vi "Dashboard Main.vi"() -> ()   [LabVIEW 2015]
uses:
  <vilib>/Utility/miscctls.llb/LVRowAndColumnTypeDef.ctl
  <vilib>/event_ctls.llb/eventvkey.ctl
  <vilib>/Rock Robotics/WPI/Dashboard/WPI_DashboardLogging Global.vi
  <vilib>/Utility/config.llb/Write Key (String).vi
  <vilib>/Utility/config.llb/Write Key (I32).vi
  <vilib>/Utility/config.llb/NI_LVConfig.lvlib
panel:
  in  "TCP":refnum<k5>
  in  "Rec Mode":enum32{"Stop", "Record", "Playback"}(radio)
  in  "Vision":u16(ring) items=["Camera Off", "USB Camera SW", "USB Camera HW", "IP Camera"]
  out "Camera IP":string
  out "Image Message":string="Timeout in Camera Communications"
  in  "Dashboard Tab":T1(tab)
  out "Velocity":dbl
  out "Centered":bool
  out "Can Hit":bool
  out "Visable Image":bool
  out "Can Fit":bool
  out "Posible Velocity":bool
  out "MotorSlide4 2":dbl(slide) scale=0.0..14.0 scale format="%#_2e"
  in  "Select Auto":string(combo)
  out "NT Connection":bool
  in  "Camera Settings":T2={"Frame Rate"=30, "Compression"=30, "Size"=1} {"Frame Rate" scale=1.0..30.0; "Size" items=["640x480", "320x240", "160x120"]}
  out "Battery":cluster{"Battery V":dbl}(graph)
  out "Mode":T3(ring)=enum."Auto Disabled"
  in  "DB Camera Config":bool
  out "fps":dbl format="%#.1g"
  out "Mbps":dbl format="%#.1g"
  out "Mbps LED":bool
  in  "Test Slider":dbl(slide) scale=0.0..100.0 scale format="%#_3g"
  in  "On/Off":bool caption="Solenoid"
  in  "Test Name":u16(ring) items=["Select the test to run..."]
  in  "Test Tree":string(tree)
  in  "Motor":cluster{"Value":dbl, "Enable":bool} {"Value" scale=-1.0..1.0 scale format="%#_3g"}
  out "Progress":T4 {"Test Progress" scale=0.0..100.0}
  in  "Rev/Fwd":cluster{"Forward":bool, "Reverse":bool}
  in  "Test Ring":u16(ring) items=["Monochrome", "Color"]
  out "Cmd Status":string
  in  "Execute Command":bool
  in  "Command Params":string[][](table)
  in  "Command Selection":i32(listbox)
  in  "CheckList":i32(listbox)=11
  out "Tree":string(tree)
  out "Camera Image":T5(plugin-control)
  out "Background":bool
  # "Battery"
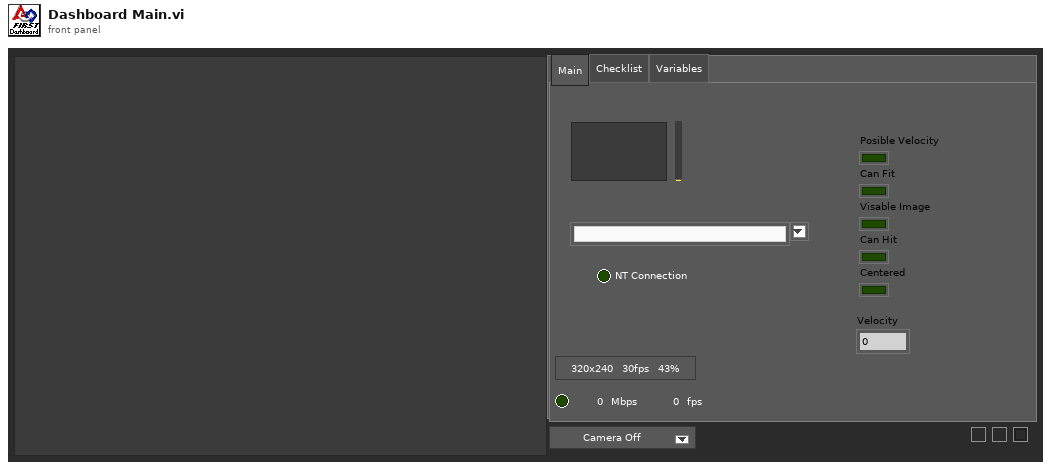
[diagram p1: front panel]
types:
  T1 = enum32{"Main", "Test", "Commands", "Checklist", "Variables"}
  T2 = cluster{"Frame Rate":i32, "Compression":i32, "Size":u16}
  T3 = enum8{"Tele-Op Disabled", "Tele-Op Enabled", "Auto Disabled", "Auto Enabled", "Test Disabled", "Test Enabled", "Disconnected", "No Code", "E-Stop"}
  T4 = cluster{"Test Progress":u8, "Test Progress Text":string}
  T5 = typedef "IMAQ Image.ctl" = refnum<image>
  T6 = cluster{"IDs":cluster{"RPC field ID":u16, "Unique ID":u16}, "String":string}
  T7 = enum32{"Drive", "Basic", "Custom", "Test", "Checklist", "Variables"}
  T8 = typedef "Image Type" = u32
  T9 = cluster{"Camera Image":refnum<vi>, "Dashboard Tab":refnum<vi>, "Background":refnum<vi>, "Vision":refnum<vi>, "Rec Mode":refnum<vi>, "Test Slider":refnum<vi>, "On/Off ":refnum<vi>, "Test Ring":refnum<vi>, "Rev/Fwd":refnum<vi>, "Test Name":refnum<vi>, "Motor":refnum<vi>, "Progress":refnum<vi>, "CheckList":refnum<vi>, "Tree":refnum<vi>, "Test Tree":refnum<vi>, "Command Params":refnum<vi>, "Command Selection":refnum<vi>, "Execute Command":refnum<vi>, "Cmd Status":refnum<vi>}
  T10 = cluster{"Error Strings":string, "Disable Counts":cluster{u16, u16}, "Rail Faults":cluster{u16, u16, u16}, "Robot IP":string, "DB Mode":u8, "Event Info":cluster{"Name":string, "Type":u8, "Number":u16, "Replay":u8}, "Camera Addr":string}
  T11 = cluster{"Status bits":cluster{"Test Mode":bool, "Autonomous":bool, "Enabled":bool, "Code Start":bool, "Brownout":bool, "Reserved 2":bool, "Reserved 3":bool, "E-Stop":bool}, "Code Trace":cluster{"Disabled":bool, "TeleOp":bool, "Auto":bool, "Test":bool}, "Controller Type":enum16{"unknown", "cRIO", "roboRio"}, "Code?":enum16{"unknown", "noCode", "code"}, "Battery V":dbl}
  T12 = cluster{"Control Bits":cluster{"TestMode":bool, "Autonomous":bool, "Enabled":bool, "FMS Present":bool, bool, bool, bool, "E-Stop":bool}, "Team Station ":u8, "Countdown":sgl, "Joystick Values":cluster{"Axes":dbl[], "Buttons":bool[], "POVs":i16[]}[]}
  T13 = typedef "NI_LVConfig.lvlib/Config Data RefNum.ctl" = refnum<k1>
  T14 = cluster{"Operation":enum16{"Update", "Clear"}, "Color Box":u32}[]
  T15 = typedef "eventvkey.ctl" = enum16{"ASCII", "Enter", "Return", "Shift", "Ctrl", "Alt", "Cmd", "Opt", "Caps", "NumLock", "Clear", "Break", "Up", "Down", "Left", "Right", "Insert", "Delete", "Home", "End", "PageUp", "PageDown", "Escape", "Help", "Pause", "ScrollLock", "F1", "F2", "F3", "F4", "F5", "F6", "F7", "F8", "F9", "F10", "F11", "F12", "F13", "F14", "F15", "F16", "F17", "F18", "F19", "F20", "F21", "F22", "F23", "F24", "Play", "VolumeUp", "VolumeDown", "Mute", "Two Byte Char"}
  T16 = cluster{"Image Size":bool, "Image Type":bool, "Pixel Value":bool, "ROI Information":bool, "Zoom Factor":bool}
  T17 = enum8{"Enabled", "Disabled", "Disabled and Grayed Out"}
  T18 = cluster{"Operation":enum16{"Update", "Clear"}, "Color Box":u32}
  T19 = typedef "LVRowAndColumnTypeDef.ctl" = cluster{"Row":i32, "Column":i32}
  T20 = cluster{"Shift":bool, "Ctrl":bool, "Alt":bool, "Cmd":bool, "Opt":bool}
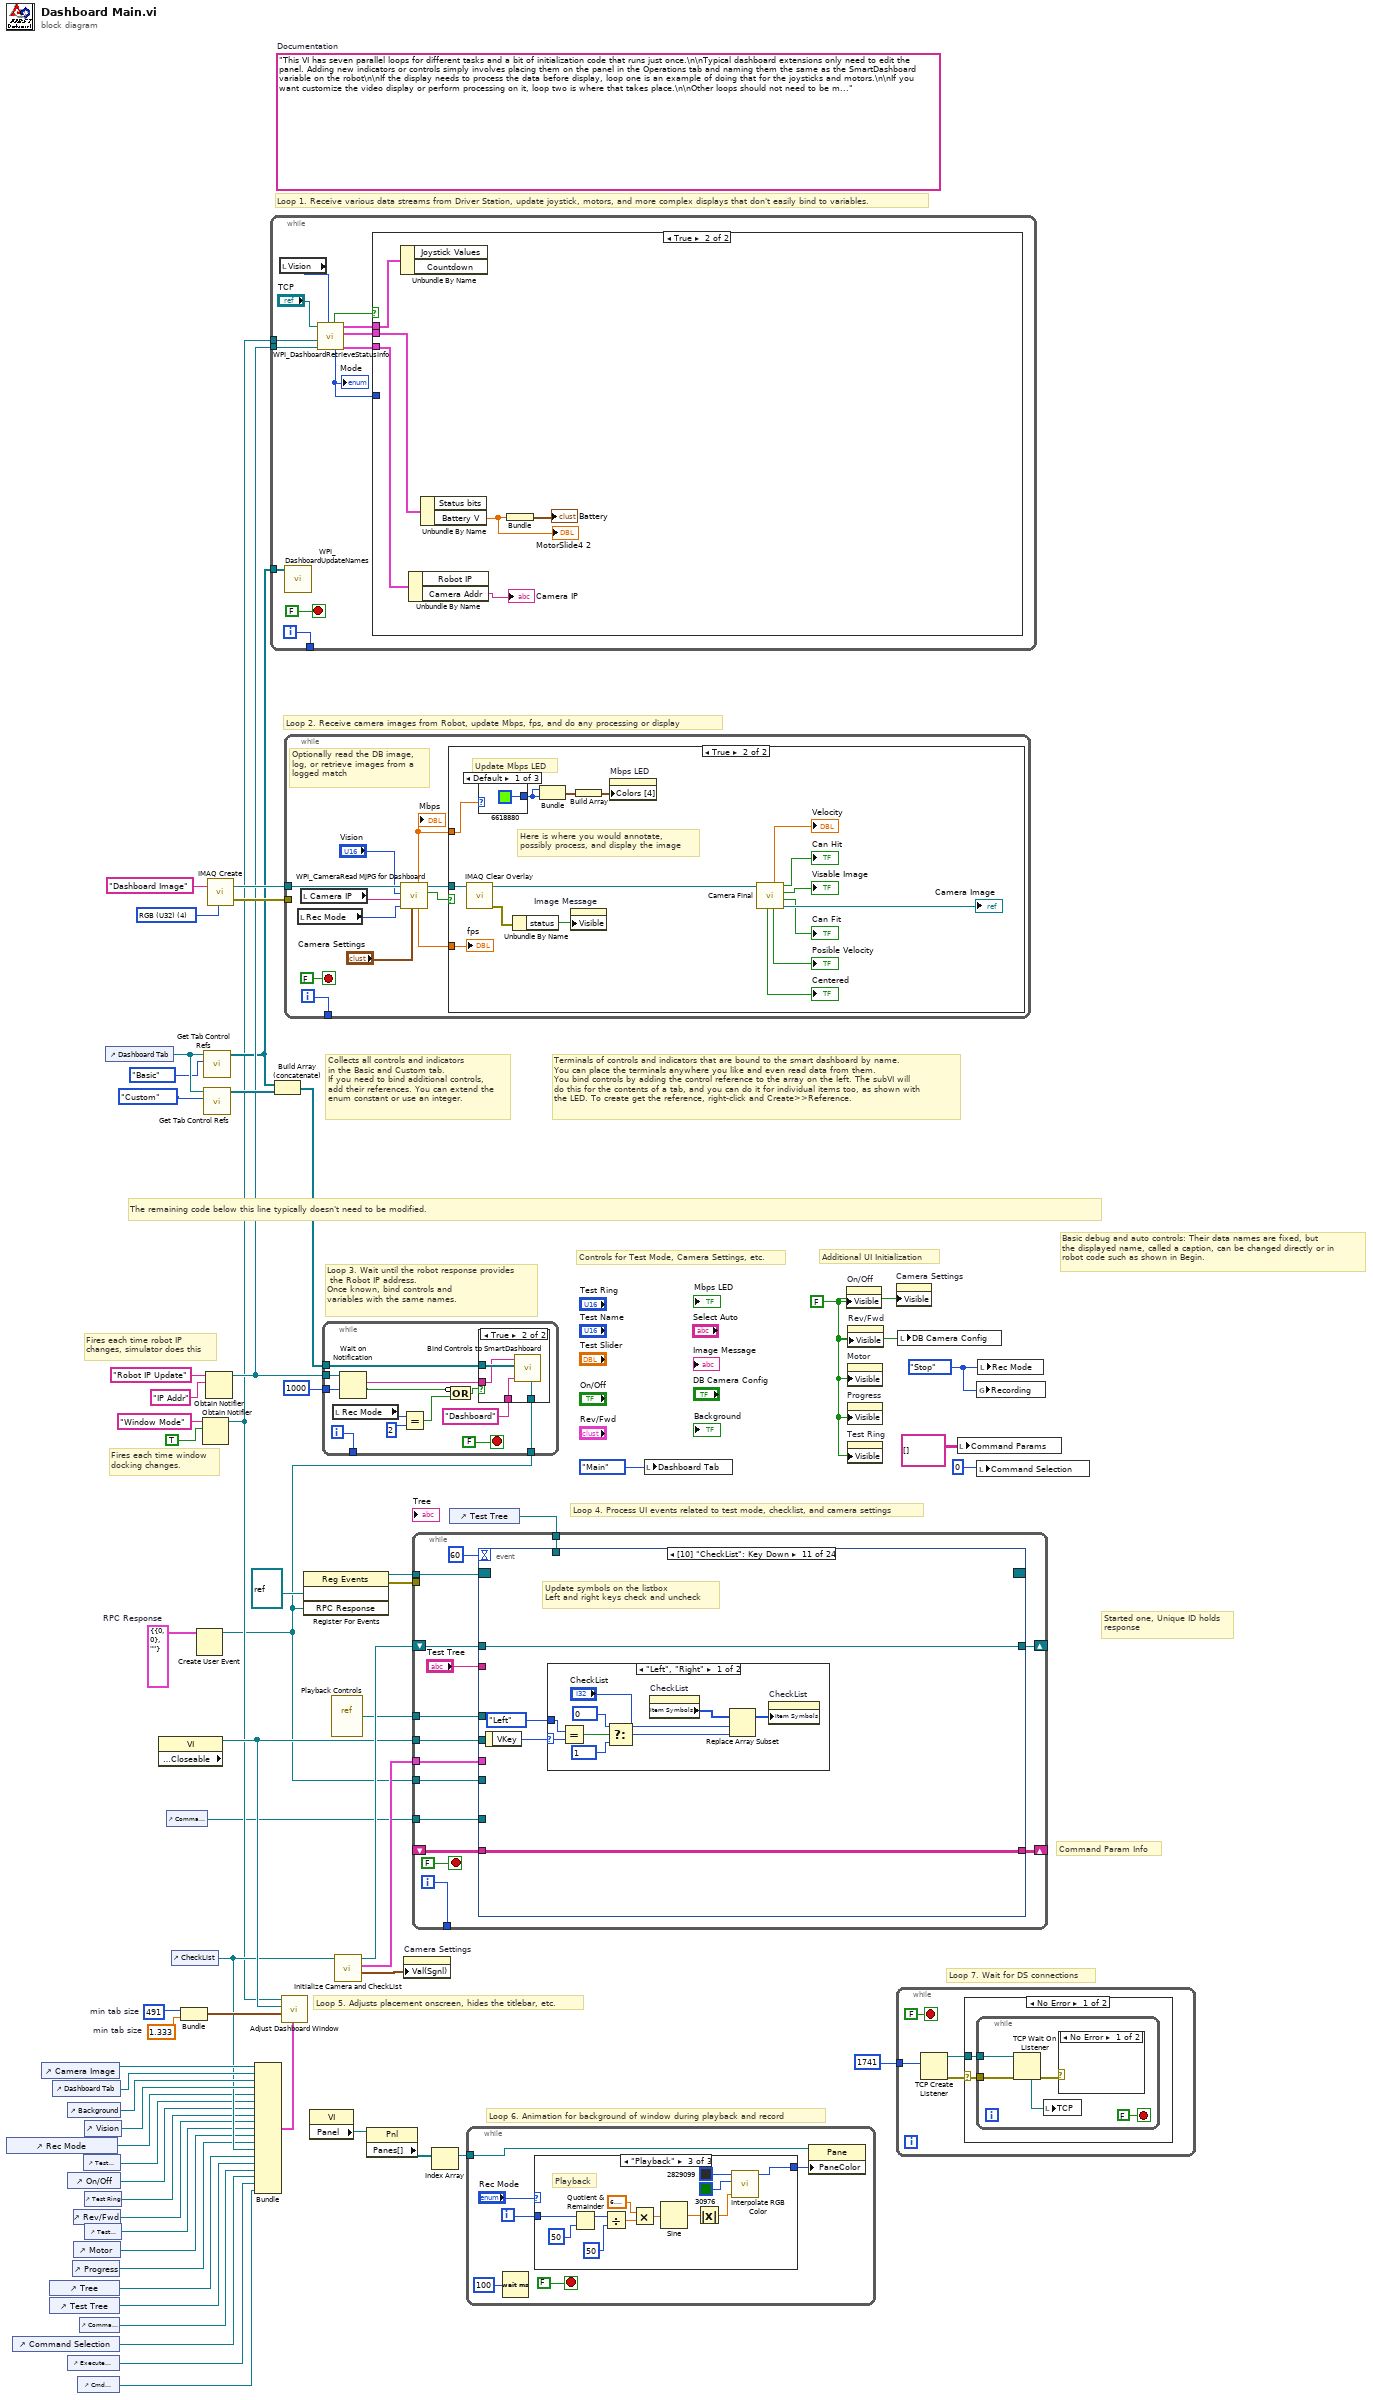
[diagram p0: block diagram]
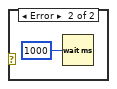
[diagram p2: hidden frame]
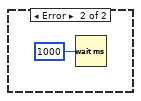
[diagram p3: hidden frame]
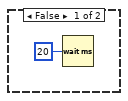
[diagram p4: hidden frame]
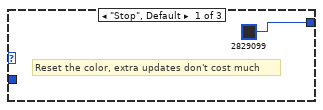
[diagram p5: hidden frame]
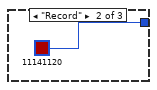
[diagram p6: hidden frame]
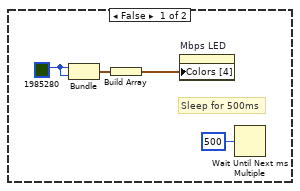
[diagram p8: hidden frame]
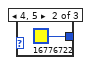
[diagram p9: hidden frame]
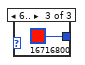
[diagram p10: hidden frame]
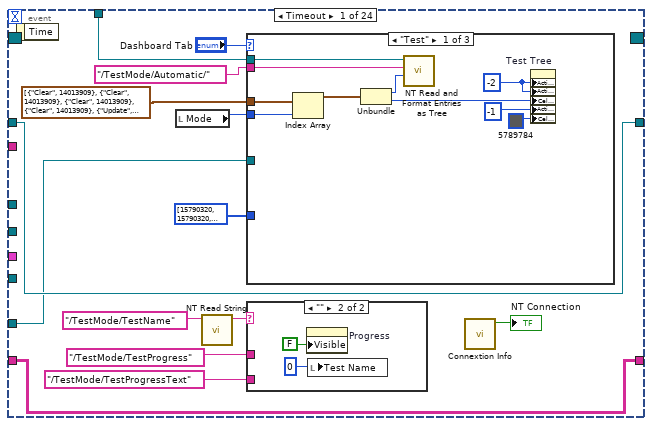
[diagram p11: hidden frame]
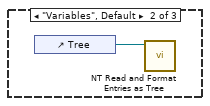
[diagram p12: hidden frame]
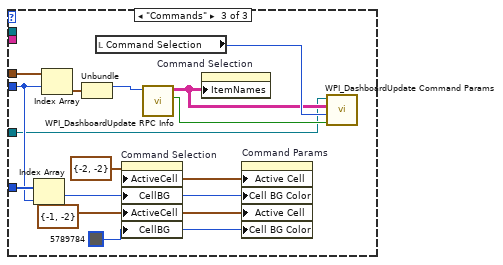
[diagram p13: hidden frame]
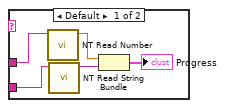
[diagram p14: hidden frame]
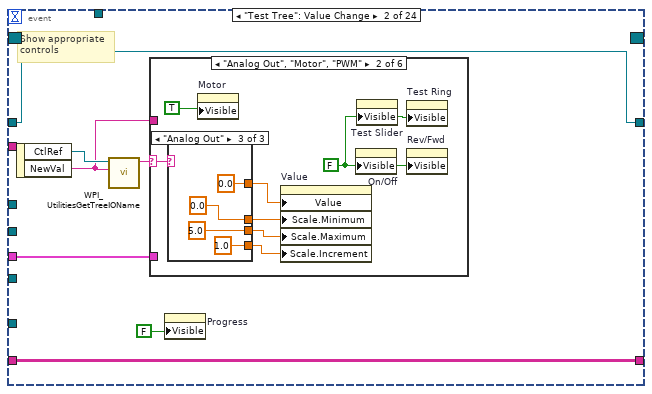
[diagram p15: hidden frame]
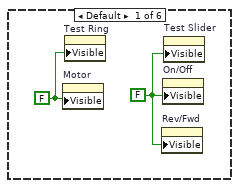
[diagram p16: hidden frame]
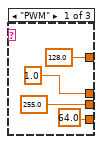
[diagram p17: hidden frame]
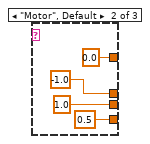
[diagram p18: hidden frame]
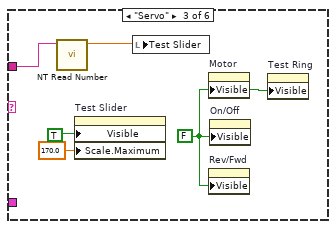
[diagram p19: hidden frame]
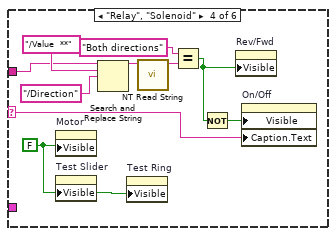
[diagram p20: hidden frame]
diagram:
  w8 = T6 {"IDs"={"RPC field ID"=0, "Unique ID"=0}, "String"=""}  # RPC Response
  w33 = 491  # min tab size
  w32 = 1.333  # min tab size
  w41 = enum32{"Stop", "Record", "Playback"}."Stop" ("Rec Mode")
  w15 = FALSE ("Visible")
  (unwired) "This VI has seven parallel loops for different tasks and a bit of initialization code that runs just once.\n\nTypical dashboard extensions only need to edit the panel. Adding new indicators or controls simply involves placing them on the panel in the Operations tab and naming them the same as the SmartDashboard variable on the robot\n\nIf the display needs to process the data before display, loop one is an example of doing that for the joysticks and motors.\n\nIf you want customize the video display or perform processing on it, loop two is where that takes place.\n\nOther loops should not need to be modified. They are pretty standard, and document the task they perform."  # Documentation
  w61 = T8 4 items=["Grayscale (U8)", "Grayscale (I16)", "Grayscale (SGL)", "Complex (CSG)", "RGB (U32)", "HSL (U32)", "RGB (U64)"] ("Image Type")
  # "Command Param Info"
  # "Started one, Unique ID holds\nresponse"
  # "Loop 7. Wait for DS connections"
  # "Basic debug and auto controls: Their data names are fixed, but\nthe displayed name, called a caption, can be changed directly or in\nrobot code such as shown in Begin."
  # "Controls for Test Mode, Camera Settings, etc."
  # "Additional UI Initialization"
  # "Loop 6. Animation for background of window during playback and record"
  # "Fires each time robot IP\nchanges, simulator does this"
  # "Fires each time window\ndocking changes."
  # "Collects all controls and indicators\nin the Basic and Custom tab.\nIf you need to bind additional controls,\nadd their references. You can extend the\nenum constant or use an integer."
  # "The remaining code below this line typically doesn't need to be modified."
  # "Loop 4. Process UI events related to test mode, checklist, and camera settings"
  # "Terminals of controls and indicators that are bound to the smart dashboard by name.\nYou can place the terminals anywhere you like and even read data from them.\nYou bind controls by adding the control reference to the array on the left. The subVI will\ndo this for the contents of a tab, and you can do it for individual items too, as shown with\nthe LED. To create get the reference, right-click and Create>>Reference."
  # "Loop 3. Wait until the robot response provides\n the Robot IP address.\nOnce known, bind controls and\nvariables with the same names."
  # "Loop 5. Adjusts placement onscreen, hides the titlebar, etc."
  # "Loop 1. Receive various data streams from Driver Station, update joystick, motors, and more complex displays that don't easily bind to variables."
  # "Loop 2. Receive camera images from Robot, update Mbps, fps, and do any processing or display"
  n1 = control-ref of="Rec Mode"() -> (w21:refnum<vi>)
  n2 = control-ref of="Command Selection"() -> (w7:refnum<vi>)
  n3 = control-ref of="Camera Image"() -> (w36:refnum<vi>)
  n4 = control-ref of="Tree"() -> (w25:refnum<vi>)
  n5 = control-ref of="Test Tree"() -> (w24:refnum<vi>)
  n6 = control-ref of="Dashboard Tab"() -> (w35:refnum<vi>)
  n7 = control-ref of="Execute Command"() -> (w9:refnum<vi>)
  n8 = control-ref of="Background"() -> (w30:refnum<vi>)
  n9 = control-ref of="On/Off"() -> (w19:refnum<vi>)
  n10 = control-ref of="Progress"() -> (w16:refnum<vi>)
  n11 = control-ref of="Rev/Fwd"() -> (w17:refnum<vi>)
  n12 = control-ref of="Motor"() -> (w22:refnum<vi>)
  n13 = control-ref of="Cmd Status"() -> (w3:refnum<vi>)
  n14 = control-ref of="Command Params"() -> (w10:refnum<vi>)
  n15 = control-ref of="Test Slider"() -> (w20:refnum<vi>)
  n16 = control-ref of="Vision"() -> (w34:refnum<vi>)
  n17 = control-ref of="Test Ring"() -> (w18:refnum<vi>)
  n18 = control-ref of="Test Name"() -> (w23:refnum<vi>)
  n19 = control-ref of="Dashboard Tab"() -> (w39:refnum<vi>)
  n20 = property class="VI" props=["Front Panel.Closeable"]() -> (reference out=w40:refnum<vi>)  [unwired: 2 in, 2 out]
  n21 = control-ref of="Command Params"() -> (w2:refnum<vi>)
  n22 = control-ref of="CheckList"() -> (w26:refnum<vi>)
  n23 = Bundle("min tab size"=w33, "min tab size"=w32) -> (w31:cluster{"min tab size":i32, "min tab size":dbl})  [unwired: 1 in]
  n24 = Create User Event(user event datatype=w8) -> (user event=w4:refnum<user-event>)  [unwired: 1 in, 1 out]
  n25 = Obtain Notifier(name (unnamed)="Window Mode", notification data type=TRUE) -> (notifier out=w12:refnum<notifier>)  [unwired: 2 in, 2 out]
  n26 = call <vilib>:"Get Tab Control Refs.vi"("Page Index"=T7."Basic" ("Dashboard Tab"), "TabControl in"=w39) -> ("ControlsOnPage"=w13:refnum<vi>[])  [unwired: 9 in]
  n27 = call <vilib>:"Get Tab Control Refs.vi"("Page Index"=T7."Custom" ("Dashboard Tab"), "TabControl in"=w39) -> ("ControlsOnPage"=w38:refnum<vi>[])  [unwired: 9 in]
  n28 = Obtain Notifier(name (unnamed)="Robot IP Update", notification data type="IP Addr" ("name (unnamed)")) -> (notifier out=w14:refnum<notifier>)  [unwired: 2 in, 2 out]
  n29 = call "IMAQ Create"("Image Name"="Dashboard Image", "Image Type"=w61) -> ("New Image"=w59:T5, "error out"=w58:errorcluster)  [unwired: 2 in, 1 out]
  n30 = Bundle("Camera Image"=w36, "Dashboard Tab"=w35, "Background"=w30, "Vision"=w34, "Rec Mode"=w21, "Test Slider"=w20, "On/Off"=w19, "Test Ring"=w18, "Rev/Fwd"=w17, "Test Name"=w23, "Motor"=w22, "Progress"=w16, "CheckList"=w26, "Tree"=w25, "Test Tree"=w24, "Command Params"=w10, "Command Selection"=w7, "Execute Command"=w9, "Cmd Status"=w3) -> (w27:T9)  [unwired: 1 in]
  n31 = while {
    tunnel: [w72] -> _
    tunnel: w14 -> [w67]
    tunnel: w13 -> [w66]
    tunnel: w12 -> [w62]
    i -> [w72]
    stop <- FALSE stop-if-true
    n32 = local read "Vision"() -> (w64:u16)
    n33 = call <vilib>:"WPI_DashboardUpdateNames.vi"("Controls on Tab"=w66) -> ()  [unwired: 11 in]
    n34 = call <vilib>:"WPI_DashboardRetrieveStatusInfo.vi"("Vision"=w64, "Binding Refnum"=w67, "Window Mode Notifier"=w62, "TCP Cnx"="TCP") -> ("Power and Errors"=w68:T10, "Status Info"=w71:T11, "Control Info"=w69:T12, "Robot Mode"=w65:T3, "Process?"=w70:bool)  [unwired: 2 in, 1 out]
    "Mode" <- w65
    n35 = case shown="True" w70 {
      tunnel: w71 -> [_ w80]
      tunnel: w69 -> [_ w79]
      tunnel: w68 -> [_ w78]
      tunnel: w65 -> [_ _]
      frame False {
        n36 = Wait (ms)(milliseconds to wait=u32 20) -> ()  [unwired: 1 out]
      }
      frame True {
        n37 = Unbundle By Name(w79) -> ()  [unwired: 2 out]
        n38 = Unbundle By Name(w78) -> ("Camera Addr"=→"Camera IP":string)  [unwired: 1 out]
        n39 = Unbundle By Name(w80) -> ("Battery V"=w75:dbl)  [unwired: 1 out]
        "MotorSlide4 2" <- w75
        n40 = Bundle("Battery V"=w75) -> (→"Battery":cluster{"Battery V":dbl})  [unwired: 1 in]
      }
    }
  }
  n41 = Build Array (concatenate)(w13, w38) -> (w37:refnum<vi>[])
  n42 = call "Adjust Dashboard Window.vi"("Sizing Refnums"=w27, "Size Constraints"=w31, "VI"=w40, "WIn Mode"=w12) -> ()  [unwired: 8 in]
  n43 = while {
    tunnel: w59 -> [w89]
    tunnel: w58 -> [_]
    tunnel: [w90] -> _
    i -> [w90]
    stop <- FALSE stop-if-true
    # "Optionally read the DB image,\nlog, or retrieve images from a\nlogged match"
    n44 = local read "Rec Mode"() -> (w84:enum32{"Stop", "Record", "Playback"})
    n45 = local read "Camera IP"() -> (w82:string)
    n46 = call <vilib>:"WPI_CameraRead MJPG for Dashboard.vi"("Camera Settings"="Camera Settings", "Rec Mode"=w84, "Camera IP"=w82, "Camera Mode"="Vision", "Refnum in"=w89) -> ("Active"=w87:bool, "Refnum out"=w88:T5, "FPS"=w86:dbl, "Bandwidth (Mbps)"=w81:dbl)  [unwired: 3 in]
    "Mbps" <- w81
    n47 = case shown="True" w87 {
      tunnel: w88 -> [_ w106]
      tunnel: w81 -> [_ w105]
      tunnel: w86 -> [_ w104]
      frame False {
        w92 = u32 1985280 ("Color Box")
        # "Sleep for 500ms"
        n48 = Bundle("Color Box"=w92, "Color Box"=w92) -> (w94:cluster{"Color Box":u32, "Color Box":u32})  [unwired: 1 out]
        n49 = Build Array(w94) -> (w93:cluster{"Color Box":u32, "Color Box":u32}[])
        n50 = property on="Mbps LED" class="Bool (strict)"("Colors [4]"=w93) -> ()  [unwired: 2 in, 2 out]
        n51 = Wait Until Next ms Multiple(millisecond multiple=u32 500) -> ()  [unwired: 1 out]
      }
      frame True {
        # "Here is where you would annotate,\npossibly process, and display the image"
        # "Update Mbps LED"
        n52 = call "IMAQ Clear Overlay"("Image"=w106) -> ("error out"=w110:errorcluster, "Image Out"=w103:T5)  [unwired: 2 in, 7 out]
        n53 = case shown="Default" w105 {
          tunnel: [u32 6618880 ("Color Box") u32 16776722 ("Color Box") u32 16716800 ("Color Box")] -> w107
          frame Default {
          }
          frame 4, 5 {
          }
          frame 6.. {
          }
        }
        n54 = Unbundle By Name(w110) -> ("status"=w111:bool)
        n55 = Bundle("Color Box"=w107, "Color Box"=w107) -> (w109:cluster{"Color Box":u32, "Color Box":u32})  [unwired: 1 out]
        n56 = property on="Image Message" class="Str"("Visible"=w111) -> ()  [unwired: 2 in, 2 out]
        n57 = Build Array(w109) -> (w108:cluster{"Color Box":u32, "Color Box":u32}[])
        n58 = property on="Mbps LED" class="Bool (strict)"("Colors [4]"=w108) -> ()  [unwired: 2 in, 2 out]
        n59 = call "Camera Final.vi"("Image Src"=w103) -> ("Image Dst Out 2"=→"Camera Image":T5, "Can Fit"=→"Can Fit":bool, "Viable Image"=→"Visable Image":bool, "Can Hit"=→"Can Hit":bool, "Possible Velocity"=→"Posible Velocity":bool, "Velocity"=→"Velocity":dbl, "Centered"=→"Centered":bool)  [unwired: 4 in]
        "fps" <- w104
      }
    }
  }
  n60 = register-events(refnum<vi> refnum, w4) -> (reference out=w45:refnum<event-registration>, error out=w44:errorcluster)  [unwired: 2 in]
  n61 = property class="VI"() -> ("Panel"=w48:refnum<vi>)  [unwired: 2 in, 2 out]
  n62 = while {
    tunnel: w37 -> [w127]
    tunnel: w14 -> [w125]
    tunnel: [w123] -> _
    tunnel: u32 1000 ("milliseconds to wait") -> [w122]
    tunnel: w4 -> [w115]
    i -> [w123]
    stop <- FALSE stop-if-true
    n63 = local read "Rec Mode"() -> (w118:enum32{"Stop", "Record", "Playback"})
    n64 = Wait on Notification(notifier=w125, timeout in ms (-1)=w122) -> (notification=w124:string, timed out?=w120:bool)  [unwired: 2 in, 2 out]
    n65 = Equal?(x=w118, y=u16 2 ("Rec Mode")) -> (x = y?=w119:bool)
    n66 = Compound Arithmetic op=OR(invert w120, w119) -> (w121:bool)
    n67 = case shown="True" w121 {
      tunnel: w127 -> [_ w131]
      tunnel: w124 -> [_ w130]
      tunnel: "Dashboard" -> [_ w129]
      tunnel: w115 -> [_ w128]
      frame False {
      }
      frame True {
        n68 = call <vilib>:"Bind Controls to SmartDashboard.vi"("RPC ref"=w128, "Client Name"=w129, "Bound Control Refs"=w131, "Server IP Address"=w130) -> ()  [unwired: 8 in]
      }
    }
  }
  n69 = vi-ref "Playback Controls.vi"() -> (w46:refnum<vi>)
  n70 = call "Initialize Camera and CheckList.vi"("ListBox in"=w26) -> ("Cluster"=w52:cluster{"value":i32, "value":i32, "index":i32}, "Array"=w53:cluster{string[]}[], "File Refnum"=w51:T13)  [unwired: 8 in]
  n71 = property class="Pnl"(reference=w48) -> ("Panes[]"=w49:refnum<vi>[])  [unwired: 1 in, 2 out]
  n72 = property on="Camera Settings" class="Clust (strict)"("Val(Sgnl)"=w52) -> ()  [unwired: 2 in, 2 out]
  n73 = Index Array(array=w49) -> (element=w47:refnum<vi>)  [unwired: 1 in]
  n74 = control-ref of="Test Tree"() -> (w50:refnum<vi>)
  n75 = while {
    tunnel: w53 -> [w143]
    shift-right: [w142] -> _
    shift-left: w51 -> [w141]
    tunnel: [w140] -> _
    tunnel: w50 -> [w139]
    tunnel: w46 -> [w138]
    tunnel: w45 -> [w137]
    tunnel: w44 -> [_]
    tunnel: w40 -> [w136]
    tunnel: w4 -> [w135]
    tunnel: w2 -> [w134]
    shift-right: [w133] -> _
    shift-left: _ -> [w132]
    i -> [w140]
    stop <- FALSE stop-if-true
    n76 = event shown="[10] \"CheckList\": Key Down" {
      selector: w137 -> [_ _ _ _ _ _ _ _ _ _ _ _ _ _ _ _ _ _ _ _ _ _ _ _]
      dyn-events: [_ _ _ _ _ _ _ _ _ _ _ _ _ _ _ _ _ _ w452 _ _ _ _ _] -> _
      timeout: u32 60 ("milliseconds to wait") -> [_ _ _ _ _ _ _ _ _ _ _ _ _ _ _ _ _ _ _ _ _ _ _ _]
      tunnel: w139 -> [w156 _ _ _ _ _ _ _ _ _ _ _ _ _ _ _ _ _ _ _ _ _ _ _]
      tunnel: "Test Tree" -> [_ _ _ _ _ _ _ _ _ _ _ _ _ w415 w424 w427 w432 w441 _ _ _ _ _ _]
      tunnel: w143 -> [_ w194 _ _ _ _ _ _ _ _ _ w377 w408 _ _ _ _ _ _ _ _ _ _ _]
      tunnel: [w153 w193 w297 w303 w313 w317 w323 w335 w343 w349 w362 w376 w401 w414 w422 w426 w431 w440 w454 w470 w472 w480 w491 w496] -> w142
      tunnel: w141 -> [w153 w193 w297 w303 w313 w317 w323 w335 w343 w349 w362 w375 w401 w414 w422 w426 w431 w440 w454 w470 w472 w480 w491 w496]
      tunnel: w138 -> [_ _ _ _ _ _ _ _ _ _ _ _ _ _ _ _ _ _ w455 _ w475 _ _ _]
      tunnel: w136 -> [_ _ _ _ _ _ _ _ _ _ _ _ _ _ _ _ _ _ w450 _ _ _ _ _]
      tunnel: w135 -> [_ _ _ _ _ _ _ _ _ _ _ _ _ _ _ _ _ _ w446 _ _ _ _ _]
      tunnel: w134 -> [w148 _ _ _ _ _ w321 _ _ _ _ _ _ _ _ _ _ _ _ _ _ _ _ _]
      tunnel: [w147 w192 w296 w302 w312 w318 w319 w329 w340 w348 w361 w374 w400 w413 w421 w425 w430 w439 w445 w468 w471 w476 w484 w497] -> w133
      tunnel: w132 -> [w147 w192 w296 w302 w312 w318 w319 _ _ w348 w361 w374 w400 w413 w421 w425 w430 w439 w445 w468 w471 w476 w484 w497]
      event Timeout {
        n77 = event-data() -> ()  [unwired: 1 in, 1 out]
        n78 = local read "Mode"() -> (w150:T3)
        n79 = call <vilib>:"NT Read String.vi"("Name"="/TestMode/TestName") -> ("String"=w159:string)  [unwired: 9 in, 1 out]
        n80 = case shown="\"Test\"" "Dashboard Tab" {
          tunnel: w156 -> [w170 _ _]
          tunnel: "/TestMode/Automatic/" ("Name Pattern") -> [w169 _ _]
          tunnel: T14 [{"Operation"=enum."Clear", "Color Box"=14013909}, {"Operation"=enum."Clear", "Color Box"=14013909}, {"Operation"=enum."Clear", "Color Box"=14013909}, {"Operation"=enum."Clear", "Color Box"=14013909}, {"Operation"=enum."Update", "Color Box"=14013909}, {"Operation"=enum."Update", "Color Box"=16777215}, {"Operation"=enum."Clear", "Color Box"=14013909}, {"Operation"=enum."Clear", "Color Box"=14013909}, {"Operation"=enum."Clear", "Color Box"=14013909}] -> [w162 _ w179]
          tunnel: w150 -> [w161 _ w178]
          tunnel: u32[] [15790320, 15790320, 15790320, 15790320, 16777215, 16777215, 15790320, 15790320, 15790320] -> [_ _ w184]
          tunnel: w148 -> [_ _ w172]
          frame "Test" {
            w168 = -2 ("Active Item:Row Number")
            n81 = Index Array(array=w162, index=w161) -> (element=w163:T18)
            n82 = Unbundle(w163) -> ("Operation"=w164:enum16{"Update", "Clear"}, "Color Box"=w165:u32)
            n83 = call <vilib>:"NT Read and Format Entries as Tree.vi"("Operation"=w164, "Name Pattern"=w169, "Tree Refnum"=w170) -> ()  [unwired: 7 in, 2 out]
            n84 = property on="Test Tree" class="Tree (strict)"("Active Item Row Number"=w168, "ActiveColNum"=w168, "CellBG"=w165, "Active Item Row Number"=-1 ("Active Item:Row Number"), "CellBG"=u32 5789784 ("Color Box")) -> ()  [unwired: 2 in, 2 out]
          }
          frame "Variables", Default {
            n85 = control-ref of="Tree"() -> (w171:refnum<vi>)
            n86 = call <vilib>:"NT Read and Format Entries as Tree.vi"("Tree Refnum"=w171) -> ()  [unwired: 9 in, 2 out]
          }
          frame "Commands" {
            w180 = u32 5789784 ("Color Box")
            w181 = T19 {"Row"=-1, "Column"=-2} ("Active Cell:Active Cell")
            w183 = T19 {"Row"=-2, "Column"=-2} ("Active Cell:Active Cell")
            n87 = Index Array(array=w184, index=w178) -> (element=w182:u32)
            n88 = Index Array(array=w179, index=w178) -> (element=w177:T18)
            n89 = Unbundle(w177) -> ("Operation"=w176:enum16{"Update", "Clear"})  [unwired: 1 out]
            n90 = local read "Command Selection"() -> (w175:i32)
            n91 = property on="Command Selection" class="MCListbox (strict)"("ActiveCell"=w183, "CellBG"=w182, "ActiveCell"=w181, "CellBG"=w180) -> ()  [unwired: 2 in, 2 out]
            n92 = call <vilib>:"WPI_DashboardUpdate RPC Info.vi"("Operation"=w176) -> ("update"=w174:bool, "commands"=w173:string[][])  [unwired: 9 in]
            n93 = property on="Command Selection" class="MCListbox (strict)"("ItemNames"=w173) -> ()  [unwired: 2 in, 2 out]
            n94 = property on="Command Params" class="Tbl (strict)"("Active Cell"=w183, "Cell BG Color"=w182, "Active Cell"=w181, "Cell BG Color"=w180) -> ()  [unwired: 2 in, 2 out]
            n95 = call <vilib>:"WPI_DashboardUpdate Command Params.vi"("Update"=w174, "NewVal"=w175, "Commands"=w173, "Param Tbl"=w172) -> ()  [unwired: 7 in, 1 out]
          }
        }
        n96 = case shown="\"\"" w159 {
          tunnel: "/TestMode/TestProgress" ("Name") -> [w186 _]
          tunnel: "/TestMode/TestProgressText" ("Name") -> [w185 _]
          frame Default {
            n97 = call <vilib>:"NT Read Number.vi"("Name"=w186) -> ("Numeric"=w187:dbl)  [unwired: 9 in, 1 out]
            n98 = call <vilib>:"NT Read String.vi"("Name"=w185) -> ("String"=w188:string)  [unwired: 9 in, 1 out]
            n99 = Bundle("Numeric"=w187, "String"=w188) -> (→"Progress":cluster{"Numeric":dbl, "String":string})  [unwired: 1 in]
          }
          frame "" {
            n100 = property on="Progress" class="Clust (strict)"("Visible"=FALSE) -> ()  [unwired: 2 in, 2 out]
            n101 = local write "Test Name"(u16 0) -> ()
          }
        }
        n102 = call <vilib>:"Connextion Info.vi"() -> ("Connected"=→"NT Connection":bool)  [unwired: 10 in, 1 out]
      }
      event "Test Tree": Value Change {
        # "Show appropriate\ncontrols"
        n103 = event-data() -> ("CtlRef"=w197:refnum<vi>, "NewVal"=w195:string)  [unwired: 1 in]
        n104 = call <vilib>:"WPI_UtilitiesGetTreeIOName.vi"("NewVal"=w195, "TreeControl in"=w197) -> ("I/O Name"=w198:string)  [unwired: 9 in]
        n105 = case shown="\"Analog Out\", \"Motor\", \"PWM\"" w198 {
          selector: w198 -> [_ w205 _ w227 w236 _]
          tunnel: w195 -> [_ _ w224 w226 _ w243]
          tunnel: w194 -> [_ _ _ _ _ w242]
          frame Default {
            w200 = FALSE ("Visible")
            w199 = FALSE ("Visible")
            n106 = property on="Motor" class="Clust (strict)"("Visible"=w199) -> ()  [unwired: 2 in, 2 out]
            n107 = property on="Test Ring" class="Ring (strict)"("Visible"=w199) -> ()  [unwired: 2 in, 2 out]
            n108 = property on="Rev/Fwd" class="Clust (strict)"("Visible"=w200) -> ()  [unwired: 2 in, 2 out]
            n109 = property on="On/Off" class="Bool (strict)"("Visible"=w200) -> ()  [unwired: 2 in, 2 out]
            n110 = property on="Test Slider" class="Slide (strict)"("Visible"=w200) -> ()  [unwired: 2 in, 2 out]
          }
          frame "Analog Out", "Motor", "PWM" {
            w206 = FALSE ("Visible")
            n111 = case shown="\"Analog Out\"" w205 {
              tunnel: [1.0 ("Value") -1.0 ("Value") 0.0 ("Value")] -> w204
              tunnel: [255.0 ("Value") 1.0 ("Value") 5.0 ("Value")] -> w203
              tunnel: [128.0 ("Value") 0.0 ("Value") 0.0 ("Value")] -> w202
              tunnel: [64.0 ("Value") 0.5 ("Value") 1.0 ("Value")] -> w201
              frame "PWM" {
              }
              frame "Motor", Default {
              }
              frame "Analog Out" {
              }
            }
            n112 = property on="Motor" class="Clust (strict)"("Visible"=TRUE) -> ()  [unwired: 2 in, 2 out]
            n113 = property on="Value" class="Slide (strict)"("Value"=w202, "Scale.Minimum"=w204, "Scale.Maximum"=w203, "Scale.Increment"=w201) -> ()  [unwired: 2 in, 2 out]
            n114 = property on="On/Off" class="Bool (strict)"("Visible"=w206) -> ()  [unwired: 2 in, 2 out]
            n115 = property on="Test Slider" class="Slide (strict)"("Visible"=w206) -> ()  [unwired: 2 in, 2 out]
            n116 = property on="Test Ring" class="Ring (strict)"("Visible"=w206) -> ()  [unwired: 2 in, 2 out]
            n117 = property on="Rev/Fwd" class="Clust (strict)"("Visible"=w206) -> ()  [unwired: 2 in, 2 out]
          }
          frame "Servo" {
            w222 = FALSE ("Visible")
            n118 = call <vilib>:"NT Read Number.vi"("Name"=w224) -> ("Numeric"=w223:dbl)  [unwired: 9 in, 1 out]
            n119 = property on="Test Slider" class="Slide (strict)"("Visible"=TRUE, "Scale.Maximum"=170.0 ("Scale.Range:Maximum")) -> ()  [unwired: 2 in, 2 out]
            n120 = local write "Test Slider"(w223) -> ()
            n121 = property on="Motor" class="Clust (strict)"("Visible"=w222) -> ()  [unwired: 2 in, 2 out]
            n122 = property on="Rev/Fwd" class="Clust (strict)"("Visible"=w222) -> ()  [unwired: 2 in, 2 out]
            n123 = property on="On/Off" class="Bool (strict)"("Visible"=w222) -> ()  [unwired: 2 in, 2 out]
            n124 = property on="Test Ring" class="Ring (strict)"("Visible"=w222) -> ()  [unwired: 2 in, 2 out]
          }
          frame "Relay", "Solenoid" {
            w225 = FALSE ("Visible")
            n125 = property on="Motor" class="Clust (strict)"("Visible"=w225) -> ()  [unwired: 2 in, 2 out]
            n126 = property on="Test Slider" class="Slide (strict)"("Visible"=w225) -> ()  [unwired: 2 in, 2 out]
            n127 = Search and Replace String(input string=w226, search string="/Value  **", replace string="/Direction") -> (result string=w232:string)  [unwired: 5 in, 3 out]
            n128 = property on="Test Ring" class="Ring (strict)"("Visible"=w225) -> ()  [unwired: 2 in, 2 out]
            n129 = call <vilib>:"NT Read String.vi"("Name"=w232) -> ("String"=w230:string)  [unwired: 9 in, 1 out]
            n130 = Equal?(x="Both directions", y=w230) -> (x = y?=w228:bool)
            n131 = Not(x=w228) -> (.not. x?=w229:bool)
            n132 = property on="Rev/Fwd" class="Clust (strict)"("Visible"=w228) -> ()  [unwired: 2 in, 2 out]
            n133 = property on="On/Off" class="Bool (strict)"("Visible"=w229, "Caption.Text"=w227) -> ()  [unwired: 2 in, 2 out]
          }
          frame "Compressor", "Digital Out" {
            w235 = FALSE ("Visible")
            # "Get direction and finish"
            n134 = property on="Motor" class="Clust (strict)"("Visible"=w235) -> ()  [unwired: 2 in, 2 out]
            n135 = property on="Test Slider" class="Slide (strict)"("Visible"=w235) -> ()  [unwired: 2 in, 2 out]
            n136 = property on="Test Ring" class="Ring (strict)"("Visible"=w235) -> ()  [unwired: 2 in, 2 out]
            n137 = property on="On/Off" class="Bool (strict)"("Visible"=TRUE, "Caption.Text"=w236) -> ()  [unwired: 2 in, 2 out]
            n138 = property on="Rev/Fwd" class="Clust (strict)"("Visible"=FALSE) -> ()  [unwired: 2 in, 2 out]
          }
          frame "Camera" {
            n139 = call <vilib>:"Get Last Path Segment.vi"("String in"=w243) -> ("String out"=w244:string)  [unwired: 10 in]
            n140 = property on="On/Off" class="Bool (strict)"("Visible"=FALSE) -> ()  [unwired: 2 in, 2 out]
            n141 = property on="Motor" class="Clust (strict)"("Visible"=FALSE) -> ()  [unwired: 2 in, 2 out]
            n142 = property on="Rev/Fwd" class="Clust (strict)"("Visible"=FALSE) -> ()  [unwired: 2 in, 2 out]
            n143 = case shown="\"White Balance  **\"" w244 {
              tunnel: w243 -> [w250 w259 w268 w277 w286 _ w292]
              tunnel: w242 -> [w248 w256 w265 w274 w283 _ _]
              frame "Size  **" {
                n144 = Index Array(array=w248) -> (element=w247:cluster{string[]})  [unwired: 1 in]
                n145 = call <vilib>:"NT Read String.vi"("Name"=w250) -> ("String"=w249:string)  [unwired: 9 in, 1 out]
                n146 = Unbundle(w247) -> (w245:string[])
                n147 = Match First String(2:w245, 3:w249) -> (0:w246:i32)  [unwired: 1 out]
                n148 = property on="Test Ring" class="Ring (strict)"("Value"=w246, "Strings []"=w245) -> ()  [unwired: 2 in, 2 out]
                n149 = property on="Test Ring" class="Ring (strict)"("Visible"=TRUE) -> ()  [unwired: 2 in, 2 out]
                n150 = property on="Test Slider" class="Slide (strict)"("Visible"=FALSE) -> ()  [unwired: 2 in, 2 out]
              }
              frame "White Balance  **" {
                n151 = Index Array(array=w256, index=1) -> (element=w257:cluster{string[]})
                n152 = call <vilib>:"NT Read String.vi"("Name"=w259) -> ("String"=w258:string)  [unwired: 9 in, 1 out]
                n153 = Unbundle(w257) -> (w254:string[])
                n154 = Match First String(2:w254, 3:w258) -> (0:w253:i32)  [unwired: 1 out]
                n155 = property on="Test Ring" class="Ring (strict)"("Value"=w253, "Strings []"=w254) -> ()  [unwired: 2 in, 2 out]
                n156 = property on="Test Ring" class="Ring (strict)"("Visible"=TRUE) -> ()  [unwired: 2 in, 2 out]
                n157 = property on="Test Slider" class="Slide (strict)"("Visible"=FALSE) -> ()  [unwired: 2 in, 2 out]
              }
              frame "Exposure  **" {
                n158 = Index Array(array=w265, index=2) -> (element=w266:cluster{string[]})
                n159 = call <vilib>:"NT Read String.vi"("Name"=w268) -> ("String"=w267:string)  [unwired: 9 in, 1 out]
                n160 = Unbundle(w266) -> (w262:string[])
                n161 = Match First String(2:w262, 3:w267) -> (0:w263:i32)  [unwired: 1 out]
                n162 = property on="Test Ring" class="Ring (strict)"("Value"=w263, "Strings []"=w262) -> ()  [unwired: 2 in, 2 out]
                n163 = property on="Test Ring" class="Ring (strict)"("Visible"=TRUE) -> ()  [unwired: 2 in, 2 out]
                n164 = property on="Test Slider" class="Slide (strict)"("Visible"=FALSE) -> ()  [unwired: 2 in, 2 out]
              }
              frame "Exposure Priority  **" {
                n165 = Index Array(array=w274, index=3) -> (element=w275:cluster{string[]})
                n166 = call <vilib>:"NT Read String.vi"("Name"=w277) -> ("String"=w276:string)  [unwired: 9 in, 1 out]
                n167 = Unbundle(w275) -> (w271:string[])
                n168 = Match First String(2:w271, 3:w276) -> (0:w272:i32)  [unwired: 1 out]
                n169 = property on="Test Ring" class="Ring (strict)"("Value"=w272, "Strings []"=w271) -> ()  [unwired: 2 in, 2 out]
                n170 = property on="Test Ring" class="Ring (strict)"("Visible"=TRUE) -> ()  [unwired: 2 in, 2 out]
                n171 = property on="Test Slider" class="Slide (strict)"("Visible"=FALSE) -> ()  [unwired: 2 in, 2 out]
              }
              frame "Color Enable  **" {
                n172 = Index Array(array=w283, index=4) -> (element=w284:cluster{string[]})
                n173 = call <vilib>:"NT Read String.vi"("Name"=w286) -> ("String"=w285:string)  [unwired: 9 in, 1 out]
                n174 = Unbundle(w284) -> (w280:string[])
                n175 = Match First String(2:w280, 3:w285) -> (0:w281:i32)  [unwired: 1 out]
                n176 = property on="Test Ring" class="Ring (strict)"("Value"=w281, "Strings []"=w280) -> ()  [unwired: 2 in, 2 out]
                n177 = property on="Test Ring" class="Ring (strict)"("Visible"=TRUE) -> ()  [unwired: 2 in, 2 out]
                n178 = property on="Test Slider" class="Slide (strict)"("Visible"=FALSE) -> ()  [unwired: 2 in, 2 out]
              }
              frame Default {
                n179 = property on="Test Ring" class="Ring (strict)"("Visible"=FALSE) -> ()  [unwired: 2 in, 2 out]
                n180 = property on="Test Slider" class="Slide (strict)"("Visible"=FALSE) -> ()  [unwired: 2 in, 2 out]
              }
              frame "Brightness  **", "Color Level  **", "Compression  **", "FPS  **", "Sharpness  **" {
                n181 = call <vilib>:"NT Read Number.vi"("Name"=w292) -> ("Numeric"=w291:dbl)  [unwired: 9 in, 1 out]
                n182 = local write "Test Slider"(w291) -> ()
                n183 = property on="Test Slider" class="Slide (strict)"("Visible"=TRUE, "Scale.Maximum"=100.0 ("Scale.Range:Maximum")) -> ()  [unwired: 2 in, 2 out]
                n184 = property on="Test Ring" class="Ring (strict)"("Visible"=FALSE) -> ()  [unwired: 2 in, 2 out]
              }
            }
          }
        }
        n185 = property on="Progress" class="Clust (strict)"("Visible"=FALSE) -> ()  [unwired: 2 in, 2 out]
      }
      event "Test Name": Mouse Enter {
        # "Populate the ring with the list of tests"
        n186 = event-data() -> ()  [unwired: 1 in, 1 out]
        n187 = call <vilib>:"NT Read String Array.vi"("Name"="/TestMode/TestList") -> ("String Array"=w301:string[])  [unwired: 9 in, 1 out]
        n188 = Build Array (concatenate)("Select the test to run...", w301) -> (w300:string[])
        n189 = property on="Test Name" class="Ring (strict)"("Strings []"=w300) -> ()  [unwired: 2 in, 2 out]
      }
      event "Test Name": Value Change {
        w304 = FALSE ("Visible")
        # "Tell the robot the test name to run"
        n190 = event-data() -> ("NewVal"=w308:u16)  [unwired: 1 in]
        n191 = property on="Test Name" class="Ring (strict)"() -> ("Strings []"=w309:string[])  [unwired: 2 in, 2 out]
        n192 = local write "Progress"(T4 {"Test Progress"=0, "Test Progress Text"=""} ("Progress")) -> ()
        n193 = Index Array(array=w309, index=w308) -> (element=w307:string)
        n194 = call <vilib>:"NT Write String.vi"("String"=w307, "Name"="/TestMode/TestName") -> ()  [unwired: 9 in, 1 out]
        n195 = property on="Progress" class="Clust (strict)"("Visible"=TRUE) -> ()  [unwired: 2 in, 2 out]
        n196 = property on="Motor" class="Clust (strict)"("Visible"=w304) -> ()  [unwired: 2 in, 2 out]
        n197 = property on="Test Slider" class="Slide (strict)"("Visible"=w304) -> ()  [unwired: 2 in, 2 out]
        n198 = property on="On/Off" class="Bool (strict)"("Visible"=w304) -> ()  [unwired: 2 in, 2 out]
        n199 = property on="Rev/Fwd" class="Clust (strict)"("Visible"=w304) -> ()  [unwired: 2 in, 2 out]
        n200 = property on="Test Ring" class="Ring (strict)"("Visible"=w304) -> ()  [unwired: 2 in, 2 out]
      }
      event "Select Auto": Mouse Enter {
        # "Populate the combo box with the list of autonomous options"
        n201 = event-data() -> ()  [unwired: 1 in, 1 out]
        n202 = call <vilib>:"NT Read String Array.vi"("Name"="Auto List") -> ("String Array"=w311:string[])  [unwired: 9 in, 1 out]
        n203 = property on="Select Auto" class="CmbBox"("Strings[]"=w311) -> ()  [unwired: 2 in, 2 out]
      }
      event "Select Auto": Value Change {
        # "User modified the Auto Selection. Write to NT variable so robot knows."
        n204 = event-data() -> ("NewVal"=w315:string)  [unwired: 1 in]
        n205 = call <vilib>:"NT Write String.vi"("String"=w315, "Name"="Auto Selector") -> ()  [unwired: 9 in, 1 out]
      }
      event "Command Selection": Value Change {
        # "Get the params and show in table"
        n206 = event-data() -> ("NewVal"=w322:i32)  [unwired: 1 in]
        n207 = property on="Command Selection" class="MCListbox (strict)"() -> ("ItemNames"=w320:string[][])  [unwired: 2 in, 2 out]
        n208 = call <vilib>:"WPI_DashboardUpdate Command Params.vi"("NewVal"=w322, "Commands"=w320, "Param Tbl"=w321) -> ()  [unwired: 8 in, 1 out]
      }
      event "Execute Command": Value Change {
        # "Started one, Unique ID holds\nresponse"
        n209 = event-data() -> ()  [unwired: 1 in, 1 out]
        n210 = property on="Command Selection" class="MCListbox (strict)"() -> ("ItemNames"=w334:string[][])  [unwired: 2 in, 2 out]
        n211 = Index Array(array=w334, index (row)="Command Selection", index (col)=0) -> (element=w332:string)
        n212 = call <vilib>:"Invoke Commands.vi"("Command Params"="Command Params", "Function Name"=w332) -> ("Params"=w328:u8, "Started"=w327:bool)  [unwired: 7 in, 1 out]
        n213 = Array Subset(array="Command Params", length (row)=w328) -> (w329:string[][])  [unwired: 3 in]
        n214 = Select(t="Executing" ("Cmd Status"), s=w327, f="" ("Cmd Status")) -> (s? t:f=→"Cmd Status":string)
      }
      event "Command Selection": Double Click {
        n215 = event-data() -> ("Row"=w344:i32)  [unwired: 1 in]
        n216 = property on="Command Selection" class="MCListbox (strict)"() -> ("ItemNames"=w347:string[][])  [unwired: 2 in, 2 out]
        n217 = local read "Command Params"() -> (w342:string[][])
        n218 = Index Array(array=w347, index (row)=w344, index (col)=0) -> (element=w345:string)
        n219 = call <vilib>:"Invoke Commands.vi"("Command Params"=w342, "Function Name"=w345) -> ("Params"=w341:u8, "Started"=w336:bool)  [unwired: 7 in, 1 out]
        n220 = Array Subset(array=w342, length (row)=w341) -> (w340:string[][])  [unwired: 3 in]
        n221 = Select(t="Executing" ("Cmd Status"), s=w336, f="" ("Cmd Status")) -> (s? t:f=w337:string)
        n222 = local write "Cmd Status"(w337) -> ()
      }
      event "CheckList": Double Click {
        # "Shift clears all"
        # "Update symbols on the listbox"
        n223 = event-data() -> ("PlatMods.Shift"=w350:bool, "Row"=w352:i32)  [unwired: 1 in]
        n224 = case shown="True" w350 {
          tunnel: w352 -> [w356 _]
          tunnel: 1 -> [w355 _]
          frame False {
            n225 = property on="CheckList" class="LstBox (strict)"() -> ("Item Symbols"=w354:i32[])  [unwired: 2 in, 2 out]
            n226 = Replace Array Subset(array=w354, new element=w355, index=w356) -> (w353:i32[])
            n227 = property on="CheckList" class="LstBox (strict)"("Item Symbols"=w353) -> ()  [unwired: 2 in, 2 out]
          }
          frame True {
            w357 = 0 ("Top Row")
            n228 = property on="CheckList" class="LstBox (strict)"() -> ("Number of Rows"=w359:u32)  [unwired: 2 in, 2 out]
            n229 = Initialize Array(0, w359) -> (w358:i32[])
            n230 = property on="CheckList" class="LstBox (strict)"("Top Row"=w357, "Value"=w357, "Item Symbols"=w358) -> ()  [unwired: 2 in, 2 out]
          }
        }
      }
      event "CheckList": Key Down {
        # "Update symbols on the listbox\nLeft and right keys check and uncheck"
        n231 = event-data() -> ("VKey"=w364:T15)  [unwired: 1 in]
        n232 = case shown="\"Left\", \"Right\"" w364 {
          selector: w364 -> [w369 _]
          tunnel: eventvkey."Left" ("VKey") -> [w367 _]
          frame "Left", "Right" {
            n233 = Equal?(x=w367, y=w369) -> (x = y?=w368:bool)
            n234 = Select(t=0, s=w368, f=1) -> (s? t:f=w370:i32)
            n235 = property on="CheckList" class="LstBox (strict)"() -> ("Item Symbols"=w373:i32[])  [unwired: 2 in, 2 out]
            n236 = Replace Array Subset(array=w373, new element=w370, index="CheckList") -> (w372:i32[])
            n237 = property on="CheckList" class="LstBox (strict)"("Item Symbols"=w372) -> ()  [unwired: 2 in, 2 out]
          }
          frame Default {
          }
        }
      }
      event "DB Camera Config": Value Change {
        # "Show or hide the cluster of controls, store in ini file"
        n238 = event-data() -> ("NewVal"=w378:bool)  [unwired: 1 in]
        n239 = case shown="False" w378 {
          tunnel: w377 -> [w387 _]
          tunnel: [w380 w398] -> w376
          tunnel: w375 -> [w379 w398]
          frame False {
            w394 = "Camera"
            w397 = FALSE ("Visible")
            n240 = local read "Camera Settings"() -> (w386:T2)
            n241 = Index Array(array=w387) -> (element=w390:cluster{string[]})  [unwired: 1 in]
            n242 = Unbundle(w386) -> ("Frame Rate"=w385:i32, "Compression"=w384:i32, "Size"=w388:u16)
            n243 = Unbundle(w390) -> (w389:string[])
            n244 = Index Array(array=w389, index=w388) -> (element=w383:string)
            n245 = call-poly <vilib>:"Write Key.vi"("section"=w394, "value"=w383, "key"="Size", "refnum"=w379) -> ("refnum out"=w396:T13)  [unwired: 2 in, 5 out]
            n246 = call-poly <vilib>:"Write Key.vi"("section"=w394, "value"=w385, "key"="FrameRate", "refnum"=w396) -> ("refnum out"=w395:T13)  [unwired: 1 in, 6 out]
            n247 = property on="Camera Settings" class="Clust (strict)"("Visible"=w397) -> ()  [unwired: 2 in, 2 out]
            n248 = local write "DB Camera Config"(w397) -> ()
            n249 = call-poly <vilib>:"Write Key.vi"("section"=w394, "value"=w384, "key"="Compression", "refnum"=w395) -> ("refnum out"=w381:T13)  [unwired: 1 in, 6 out]
            n250 = call <vilib>:"Close Config Data.vi"("refnum"=w381) -> ("file path"=w382:path)  [unwired: 2 in, 8 out]
            n251 = call <vilib>:"Open Config Data.vi"("configuration file path"=w382) -> ("refnum"=w380:T13)  [unwired: 8 in, 2 out]
          }
          frame True {
            n252 = property on="Camera Settings" class="Clust (strict)"("Visible"=TRUE) -> ()  [unwired: 2 in, 2 out]
          }
        }
      }
      event "Camera Settings": Value Change {
        # "Update summary string when any elements of DB camera change"
        n253 = event-data() -> ("NewVal"=w412:T2)  [unwired: 1 in]
        n254 = Index Array(array=w408) -> (element=w407:cluster{string[]})  [unwired: 1 in]
        n255 = Unbundle(w412) -> ("Frame Rate"=w403:i32, "Compression"=w402:i32, "Size"=w405:u16)
        n256 = Unbundle(w407) -> (w406:string[])
        n257 = Index Array(array=w406, index=w405) -> (element=w404:string)
        n258 = Format Into String(format string="%s   %dfps   %d%%", w404, w403, w402) -> (resulting string=w409:string)  [unwired: 2 in, 1 out]
        n259 = Build Array(w409) -> (w410:string[])
        n260 = property on="DB Camera Config" class="Bool (strict)"("Strings [4]"=w410) -> ()  [unwired: 2 in, 2 out]
      }
      event "Motor.Enable": Value Change {
        # "When the test mode otor enable helper is set, update that\ntree row item's value"
        n261 = event-data() -> ("NewVal"=w419:bool)  [unwired: 1 in]
        n262 = Unbundle("Motor") -> ("Value"=w418:dbl)  [unwired: 1 out]
        n263 = Select(t=w418, s=w419, f=0.0) -> (s? t:f=w416:dbl)
        n264 = call <vilib>:"NT Write Number.vi"("Numeric"=w416, "Name"=w415) -> ()  [unwired: 9 in, 1 out]
      }
      event "Test Slider": Value Change {
        # "When the test mode slider helper is set, update that\ntree row item's value"
        n265 = event-data() -> ("NewVal"=w423:dbl)  [unwired: 1 in]
        n266 = call <vilib>:"NT Write Number.vi"("Numeric"=w423, "Name"=w424) -> ()  [unwired: 9 in, 1 out]
      }
      event "On/Off": Value Change {
        # "When the test mode on/off helper value is set, update that\ntree row item's value"
        n267 = event-data() -> ("NewVal"=w429:bool)  [unwired: 1 in]
        n268 = Boolean To (0,1)(Boolean=w429) -> (0, 1=w428:i16)
        n269 = call <vilib>:"NT Write Number.vi"("Numeric"=w428, "Name"=w427) -> ()  [unwired: 9 in, 1 out]
      }
      event "Rev/Fwd": Value Change {
        # "When the test mode helper value for relays is set, update that\ntree row item's value"
        n270 = event-data() -> ("NewVal.Forward"=w438:bool, "NewVal.Reverse"=w437:bool)  [unwired: 1 in]
        n271 = Boolean To (0,1)(Boolean=w438) -> (0, 1=w434:i16)
        n272 = Boolean To (0,1)(Boolean=w437) -> (0, 1=w436:i16)
        n273 = Negate(x=w436) -> (-x=w435:i16)
        n274 = Add(x=w434, y=w435) -> (x+y=w433:i16)
        n275 = call <vilib>:"NT Write Number.vi"("Numeric"=w433, "Name"=w432) -> ()  [unwired: 9 in, 1 out]
      }
      event "Test Ring": Value Change {
        # "When a test mode helper value is selected from the ring,\nset the tree item's variable to the string value"
        n276 = event-data() -> ("NewVal"=w443:u16)  [unwired: 1 in]
        n277 = property on="Test Ring" class="Ring (strict)"() -> ("Strings []"=w444:string[])  [unwired: 2 in, 2 out]
        n278 = Index Array(array=w444, index=w443) -> (element=w442:string)
        n279 = call <vilib>:"NT Write String.vi"("String"=w442, "Name"=w441) -> ()  [unwired: 9 in, 1 out]
      }
      event "Rec Mode": Value Change {
        # "Update globals for recording mode and path to read log from.\nClear when logging and let NetworkTables set path for vision to\nuse."
        n280 = event-data() -> ("NewVal"=w456:enum32{"Stop", "Record", "Playback"})  [unwired: 1 in]
        n281 = global write "WPI_DashboardLogging Global.vi" "Logging Filename"(path "") -> ()
        n282 = global write "WPI_DashboardLogging Global.vi" "Recording"(w456) -> ()
        n283 = case shown="\"Playback\"" w456 {
          tunnel: w455 -> [_ w458 w467]
          tunnel: [_ _ w466] -> w452
          tunnel: [_ _ w465] -> _
          tunnel: w450 -> [_ _ w463]
          tunnel: cluster{i32, i32} {-250, 170} -> [_ _ w462]
          tunnel: [_ _ T16 {"Image Size"=TRUE, "Image Type"=TRUE, "Pixel Value"=TRUE, "ROI Information"=TRUE, "Zoom Factor"=FALSE} ("Image Information Shown:All Elements")] -> w448
          tunnel: [_ _ TRUE ("Zoom Factor")] -> w447
          tunnel: w446 -> [_ _ w459]
          frame Default {
          }
          frame "Stop", "Record" {
            # "Place Window too"
            n284 = invoke class="VI" method="FP.Close"(reference=w458) -> (reference out=w457:refnum<vi>)  [unwired: 2 in, 2 out]
            n285 = invoke class="VI" method="Abort VI"(reference=w457) -> ()  [unwired: 2 in, 3 out]
          }
          frame "Playback" {
            n286 = call "Open Playback Panel.vi"("Offset"=w462, "DB VI Ref"=w463, "Playback in"=w467) -> ("Playback out"=w464:refnum<vi>)  [unwired: 8 in]
            n287 = register-events(w464, w459) -> (reference out=w466:refnum<event-registration>, error out=w465:errorcluster)  [unwired: 2 in]
          }
        }
        n288 = property on="Camera Image" class="ImageControl"("Image Information Shown"=w448, "Image Information Visible"=w447) -> ()  [unwired: 2 in, 2 out]
        n289 = call <vilib>:"WPI_DashboardNT Log FieldName Cache.vi"("Operation"=enum16{"Lookup/Add", "Index", "Clear"}."Clear") -> ()  [unwired: 8 in, 3 out]
      }
      event Panel Close {
        w469 = enum32{"Stop", "Record", "Playback"}."Stop" ("Rec Mode")
        # "Playback window has been closed, abort"
        n290 = event-data() -> ()  [unwired: 1 in, 4 out]
        n291 = local write "Rec Mode"(w469) -> ()
        n292 = global write "WPI_DashboardLogging Global.vi" "Recording"(w469) -> ()
      }
      event Panel Close {
        # "Abort playback window and ourself"
        n293 = event-data() -> ()  [unwired: 1 in, 4 out]
        n294 = invoke class="VI" method="FP.Close"(reference=w475) -> (reference out=w474:refnum<vi>)  [unwired: 2 in, 2 out]
        n295 = invoke class="VI" method="Abort VI"(reference=w474) -> (error out=w473:errorcluster)  [unwired: 2 in, 2 out]
        n296 = invoke class="VI" method="Abort VI"(error in=w473) -> ()  [unwired: 2 in, 3 out]
      }
      event User Event {
        n297 = event-data() -> ("IDs"=w483:cluster{"RPC field ID":u16, "Unique ID":u16}, "String"=w482:string)  [unwired: 1 in]
        n298 = Bundle("IDs"=w483, "String"=w482) -> (w481:T6)  [unwired: 1 in]
        n299 = call <vilib>:"Retrieve RPC Response.vi"("RPC Response"=w481) -> ("Output"=w478:string[][])  [unwired: 10 in]
        n300 = Build Array (concatenate)(w476, w478) -> (w477:string[][])
        n301 = local write "Command Params"(w477) -> ()
        n302 = local write "Cmd Status"("" ("Cmd Status")) -> ()
      }
      event "Vision": Value Change {
        # "Enable/Disable Compression slider.\nHW USB is hard-coded into the camera"
        n303 = event-data() -> ("NewVal"=w490:u16)  [unwired: 1 in]
        n304 = Equal?(x=w490, y=u32 2 ("milliseconds to wait")) -> (x = y?=w488:bool)
        n305 = Select(t=T17."Disabled and Grayed Out" ("Disabled"), s=w488, f=T17."Enabled" ("Disabled")) -> (s? t:f=w485:T17)
        n306 = property on="Compression" class="Slide (strict)"("DisabledEnum"=w485) -> ()  [unwired: 2 in, 2 out]
      }
      event "Tree": Double Click {
        n307 = event-data() -> ("PlatMods"=w495:T20, "Tag"=w494:string)  [unwired: 1 in]
        n308 = Unbundle(w495) -> ("Shift"=w493:bool)  [unwired: 4 out]
        n309 = Not(x=w493) -> (.not. x?=w492:bool)
        n310 = call <vilib>:"NT Update Persistence.vi"("Persistence"=w492, "Name"=w494) -> ()  [unwired: 9 in, 1 out]
      }
    }
  }
  n311 = while {
    tunnel: w47 -> [w499]
    i -> [w502]
    stop <- FALSE stop-if-true
    n312 = Wait (ms)(milliseconds to wait=u32 100) -> ()  [unwired: 1 out]
    n313 = case shown="\"Playback\"" "Rec Mode" {
      tunnel: w502 -> [_ _ w517]
      tunnel: [u32 2829099 ("Base Color") u32 11141120 ("Target Color") w506] -> w498
      frame "Stop", Default {
        # "Reset the color, extra updates don't cost much"
      }
      frame "Record" {
      }
      frame "Playback" {
        # "Playback"
        n314 = Quotient & Remainder(x=w517, y=u32 50 ("milliseconds to wait")) -> (x-y*floor(x/y)=w513:u32)  [unwired: 1 out]
        n315 = Divide(x=w513, y=u32 50 ("milliseconds to wait")) -> (x/y=w510:dbl)
        n316 = Multiply(x=6.283185307179586, y=w510) -> (x*y=w515:dbl)
        n317 = Sine(x=w515) -> (sin(x)=w514:dbl)
        n318 = Absolute Value(x=w514) -> (abs(x)=w507:dbl)
        n319 = call "Interpolate RGB Color.vi"("Proportion"=w507, "Target Color"=u32 30976, "Base Color"=u32 2829099) -> ("Result Color"=w506:u32)  [unwired: 8 in]
      }
    }
    n320 = property class="Pane"(reference=w499, "PaneColor"=w498) -> ()  [unwired: 1 in, 2 out]
  }
  n321 = local write "Dashboard Tab"(T1."Main" ("Dashboard Tab")) -> ()
  n322 = property on="On/Off" class="Bool (strict)"("Visible"=w15) -> ()  [unwired: 2 in, 2 out]
  n323 = property on="Motor" class="Clust (strict)"("Visible"=w15) -> ()  [unwired: 2 in, 2 out]
  n324 = property on="Progress" class="Clust (strict)"("Visible"=w15) -> ()  [unwired: 2 in, 2 out]
  n325 = property on="Test Ring" class="Ring (strict)"("Visible"=w15) -> ()  [unwired: 2 in, 2 out]
  n326 = property on="Rev/Fwd" class="Clust (strict)"("Visible"=w15) -> ()  [unwired: 2 in, 2 out]
  n327 = property on="Camera Settings" class="Clust (strict)"("Visible"=w15) -> ()  [unwired: 2 in, 2 out]
  n328 = while {
    tunnel: u16 1741 ("timeout ms (25000)") -> [w519]
    stop <- FALSE stop-if-true
    n329 = TCP Create Listener(10:w519) -> (0:w518:errorcluster, 3:w520:refnum<k5>)  [unwired: 4 in, 1 out]
    n330 = case shown="No Error" w518 {
      selector: w518 -> [w522 _]
      tunnel: w520 -> [w523 _]
      frame No Error {
        n331 = while {
          tunnel: w523 -> [w526]
          tunnel: w522 -> [w525]
          stop <- FALSE stop-if-true
          n332 = TCP Wait On Listener(8:w525, 11:w526) -> (0:w527:errorcluster, 4:w528:refnum<k5>)  [unwired: 2 in, 3 out]
          n333 = local write "TCP"(w528) -> ()
          n334 = case shown="No Error" w527 {
            frame No Error {
            }
            frame Error {
              n335 = Wait (ms)(milliseconds to wait=u32 1000) -> ()  [unwired: 1 out]
            }
          }
        }
      }
      frame Error {
        n336 = Wait (ms)(milliseconds to wait=u32 1000) -> ()  [unwired: 1 out]
      }
    }
  }
  n337 = local write "DB Camera Config"(w15) -> ()
  n338 = local write "Command Params"(string[][] [] ("Command Params")) -> ()
  n339 = global write "WPI_DashboardLogging Global.vi" "Recording"(w41) -> ()
  n340 = local write "Command Selection"(u16 0 ("milliseconds to wait")) -> ()
  n341 = local write "Rec Mode"(w41) -> ()
